vi "Bang-Bang Gain Tool.vi"() -> ()   [LabVIEW 2018]
doc: "This example demonstrates how to use Advanced PID autotuning VI where you can change the autotuning algorithm while you run the VI."
uses:
  <vilib>/DAQmx/read.llb/DAQmx Read (Analog DBL 1Chan 1Samp).vi
  <vilib>/DAQmx/write.llb/DAQmx Write (Analog DBL 1Chan 1Samp).vi
  <vilib>/DAQmx/create/channels.llb/DAQmx Create Channel (AO-Voltage-Basic).vi
  <vilib>/DAQmx/create/channels.llb/DAQmx Create Channel (AI-Temperature-Thermocouple).vi
  <vilib>/addons/control/pid/pid.llb/PID Gain Schedule (DBL).vi
  <vilib>/DAQmx/miscellaneous.llb/DAQmx Fill In Error Info.vi
  <vilib>/addons/control/pid/autopid.llb/PID Online Autotuning (Step Closed Loop).vi
  <vilib>/addons/control/pid/pid.llb/PID Advanced (DBL).vi
  <vilib>/addons/control/pid/NI_PID_autopid.lvlib
  <vilib>/addons/control/pid/NI_PID_pid.lvlib
  <vilib>/ptbypt/NI_PtbyPt.lvlib
panel:
  out "Numeric":dbl
  out "Heaters":bool
  in  "ON/OFF":bool caption="Heater Power"
  in  "Tab Control 2":enum32{"Instructions", "Plant Parameters"}(tab)
  in  "Instructions":string="Overview: This example demonstrates how to use the  PID Online Autotuning VI with the PID using the Closed-Loop Step Response Technique. This VI also shows how to handle Gain-scheduling process.\nInstructions:\n1. Run the VI and wait until the process variable (PV) reaches near setpoint (SP).\n2.  On the PID Autotuning Design section, select the type of controller and excitation amplitude for the 'closed-loop step response'. Then, click Autotune to start the process.\n3.  When the tuned PID gains do not change anymore, the identification is done and you can add a new gain by pressing Insert gains. That will also transfer the new gain to PID Gains array. Press Replace gains if you just want to substitute the previous recorded gains.\n4. Click Autotune again to go back to the automatic control. Look at the Gain Scheduling tab to see the new gain added to the list. You can change the plant to another setpoint and repeat this process to identify the gain for another operating point.\n5. Click Stop to stop the VI.\n"
  in  "Insert gains":bool
  in  "Tab Control":enum32{"PID", "Gain Scheduling"}(tab)
  out "PID Gains":T1={"proportional gain (Kc)"=6.925505792902687, "integral time (Ti, min)"=0.004930412653813362, "derivative time (Td, min)"=0.0} {"derivative time (Td, min)" format="%#.6g"; "integral time (Ti, min)" format="%#.6g"; "proportional gain (Kc)" format="%#.6g"}
  in  "SP:":dbl(slide)=10.0 min=0.0 max=0.0 scale=0.0..100.0
  in  "MV:":dbl(slide)=-7.438794336301588e-06 scale=-100.0..100.0
  out "PV:":dbl(slide)=45.098041757771064 scale=0.0..100.0
  in  "Autotune":bool
  in  "Reinitialize":bool
  in  "Automatic":bool=TRUE
  in  "alpha":dbl=nan format="%.2f"
  out "Gain Scheduling":i32
  in  "PID gain schedule":T2(array[cluster])=[{"PID gains"={"Kc"=7.0, "Ti"=0.001, "Td"=0.0}, "max value"=0.0}] {"max value" format="%.2f"; "PID gains"."Td" format="%#.3g"; "PID gains"."Ti" format="%#.3g"; "PID gains"."Kc" format="%#.3g"}
  in  "autotuning parameters":T3={"Type of Controller"=1, "relay cycles"=3, "amplitude"=1.0, "control specifications"=2, "PV noise level"=0.1} {"PV noise level" format="%.2f"; "control specifications" items=["fast", "normal", "slow"]; "amplitude" format="%.2f"; "Type of Controller" items=["P", "PI", "PID"]}
  out "MV":dbl(graph)
  in  "Replace gains":bool
  out "tuned PID gains":T1={"proportional gain (Kc)"=1.9838195929127882, "integral time (Ti, min)"=0.01995856284686879, "derivative time (Td, min)"=0.0} {"derivative time (Td, min)" format="%#.6g"; "integral time (Ti, min)" format="%#.6g"; "proportional gain (Kc)" format="%#.6g"}
  in  "Sampling Time dt (s)":dbl=0.05 min=0.001 step=0.01 format="%#.3p"
  in  "Stop":bool
  out "SP and PV":cluster{"initial PV":dbl, "SP1:":dbl}(graph)={"initial PV"=50.98160323470328, "SP1:"=50.98039215686275}
  # "PID Autotuning Design"
  # "Plant Simulated Parameters"
  # "Proportional-Integral-Derivative (PID) Controller"
  # "PID Gains"
  # "Operating Point"
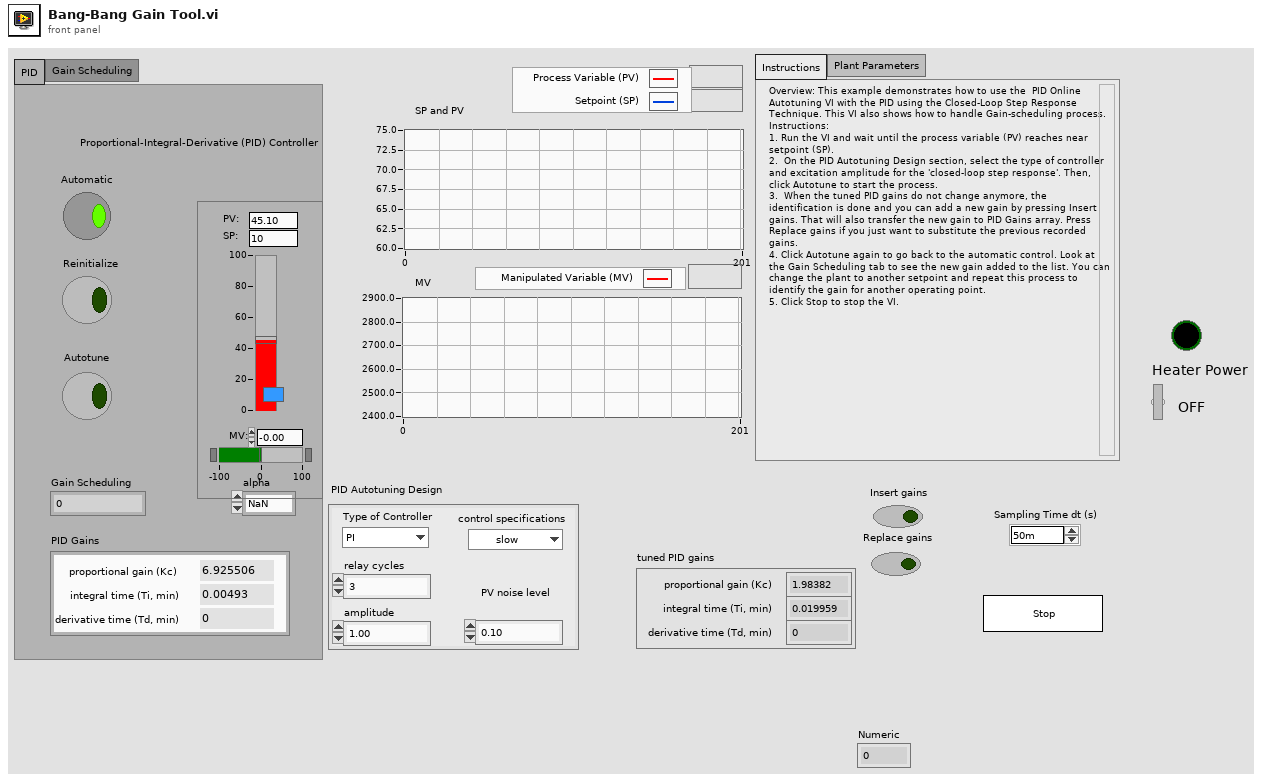
[diagram p1: front panel]
types:
  T1 = cluster{"proportional gain (Kc)":dbl, "integral time (Ti, min)":dbl, "derivative time (Td, min)":dbl}
  T2 = cluster{"PID gains":cluster{"Kc":dbl, "Ti":dbl, "Td":dbl}, "max value":dbl}[]
  T3 = cluster{"Type of Controller":u16, "relay cycles":i32, "amplitude":dbl, "control specifications":u16, "PV noise level":dbl}
  T4 = cluster{"tuned PID gains":cluster{"proportional gain (Kc)":dbl, "integral time (Ti, min)":dbl, "derivative time (Td, min)":dbl}, "SP:":dbl}
  T5 = cluster{"PID gains":cluster{"Kc":dbl, "Ti":dbl, "Td":dbl}, "max value":dbl}
  T6 = cluster{"tuned PID gains":cluster{"proportional gain (Kc)":dbl, "integral time (Ti, min)":dbl, "derivative time (Td, min)":dbl}, "max value":dbl}
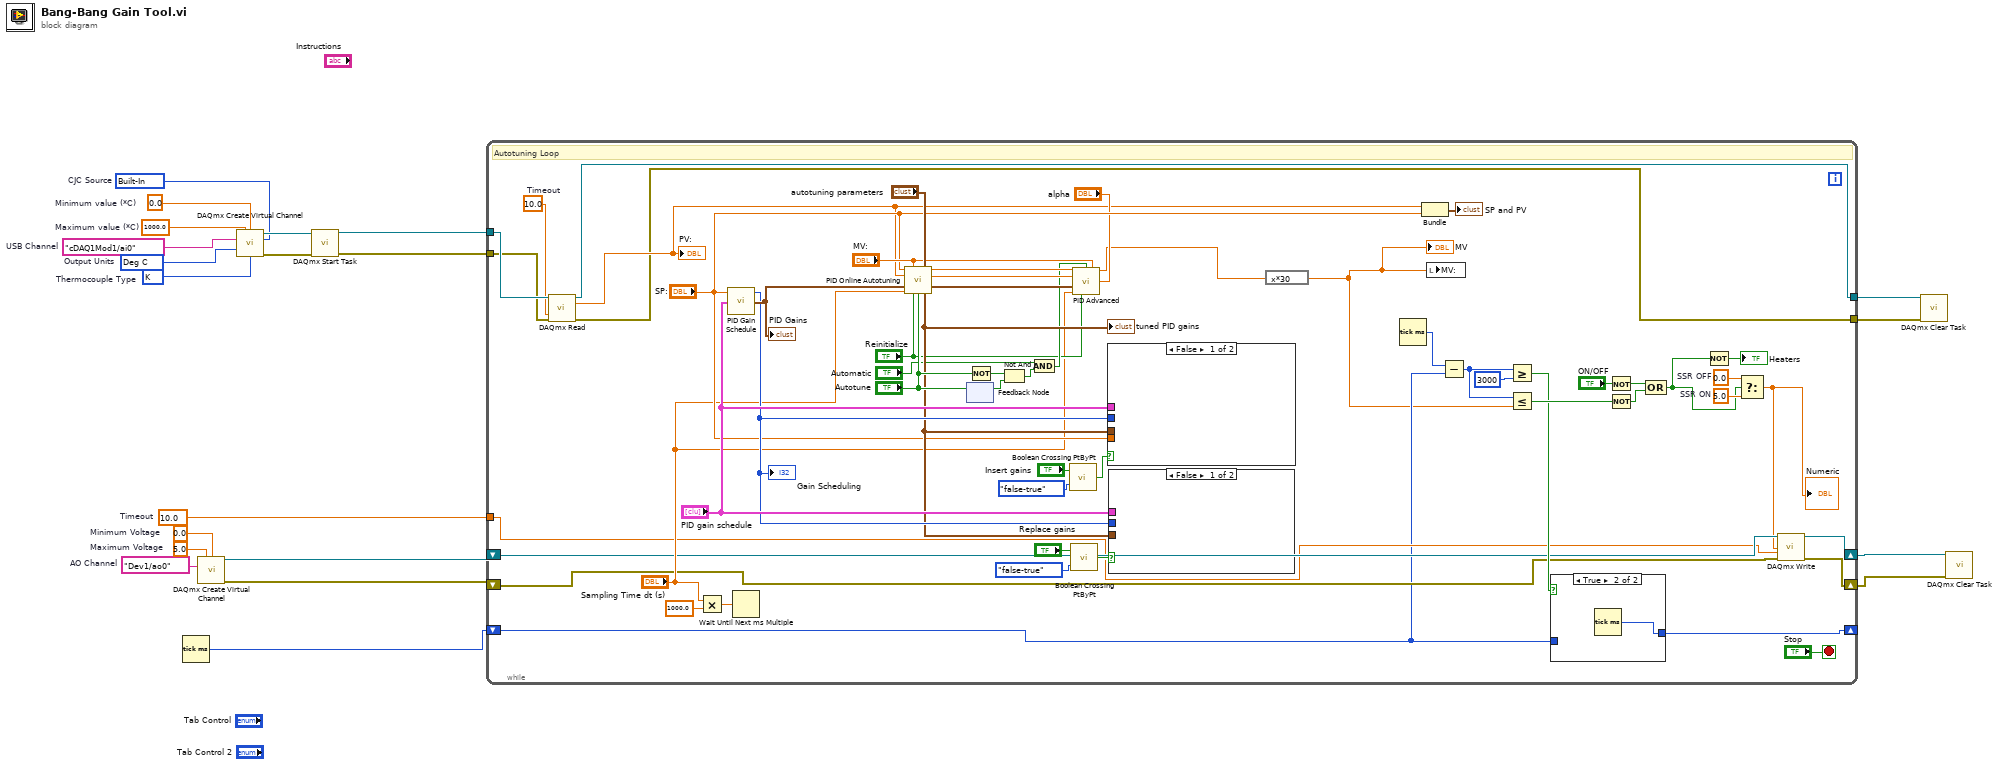
[diagram p0: block diagram]
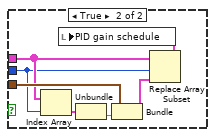
[diagram p3: hidden frame]
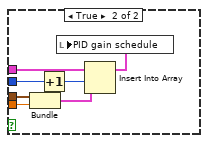
[diagram p4: hidden frame]
diagram:
  w10 = 10143 items=["Deg C"=10143, "Deg F"=10144, "Kelvins"=10325, "Deg R"=10145, "From Custom Scale"=10065]  # Output Units
  w8 = 10073 items=["J"=10072, "K"=10073, "N"=10077, "R"=10082, "S"=10085, "T"=10086, "B"=10047, "E"=10055]  # Thermocouple Type
  w9 = tag "cDAQ1Mod1/ai0"  # USB Channel
  w13 = 1000.0  # Maximum value (*C)
  w14 = 0.0  # Minimum value (*C)
  w7 = 10200 items=["Built-In"=10200, "Constant Value"=10116, "Channel"=10113]  # CJC Source
  w18 = tag "Dev1/ao0"  # AO Channel
  w19 = 5.0  # Maximum Voltage
  w20 = 0.0  # Minimum Voltage
  w15 = 10.0  # Timeout
  n1 = Tick Count (ms)() -> (millisecond timer value=w21:u32)
  n2 = call-poly <vilib>:"DAQmx Create Virtual Channel.vi"("maximum value"=w19, "minimum value"=w20, "physical channels"=w18) -> ("task out"=w17:refnum<k21>, "error out"=w16:errorcluster)  [unwired: 11 in]
  n3 = call-poly <vilib>:"DAQmx Create Virtual Channel.vi"("maximum value"=w13, "minimum value"=w14, "physical channels"=w9, "cjc source"=w7, "units"=w10, "thermocouple type"=w8) -> ("task out"=w12:refnum<k21>, "error out"=w11:errorcluster)  [unwired: 8 in]
  n4 = call <vilib>:"DAQmx Start Task.vi"("task/channels in"=w12, "error in"=w11) -> ("task out"=w6:refnum<k21>, "error out"=w5:errorcluster)  [unwired: 12 in]
  n5 = while {
    shift-right: [w38] -> _
    shift-left: w21 -> [w30]
    shift-right: [w34] -> w2
    shift-left: w17 -> [w37]
    shift-right: [w33] -> w1
    shift-left: w16 -> [w36]
    tunnel: w15 -> [w35]
    tunnel: w6 -> [w28]
    tunnel: w5 -> [w27]
    tunnel: [w25] -> w4
    tunnel: [w24] -> w3
    stop <- "Stop" stop-if-true
    w26 = 10.0  # Timeout
    w46 = 5.0  # SSR ON
    w47 = 0.0  # SSR OFF
    # "Autotuning Loop"
    n6 = call-poly <vilib>:"DAQmx Read.vi"("task/channels in"=w28, "timeout"=w26, "error in"=w27) -> ("task out"=w25:refnum<k21>, "data"=w29:dbl, "error out"=w24:errorcluster)  [unwired: 10 in]
    "PV:" <- w29
    n7 = Multiply(x="Sampling Time dt (s)", y=1000.0) -> (x*y=w55:dbl)
    n8 = call-poly <vilib>:"PID Gain Schedule.vi"("PID gain schedule"="PID gain schedule", "gain scheduling value"="SP:") -> ("PID gains out"=w65:T1, "index out"=w60:i32)  [unwired: 2 in]
    "PID Gains" <- w65
    "Gain Scheduling" <- w60
    n9 = Wait Until Next ms Multiple(millisecond multiple=w55) -> ()  [unwired: 1 out]
    n10 = call-poly <vilib>:"PID Online Autotuning.vi"("setpoint"="SP:", "manipulated variable"="MV:", "autotuning parameters"="autotuning parameters", "process variable"=w29, "PID gains in"=w65, "dt (s)"="Sampling Time dt (s)", "reinitialize? (F)"="Reinitialize", "autotune? (F)"="Autotune") -> ("setpoint out"=w76:dbl, "process variable out"=w75:dbl, "PID gains out"=w73:T1, "tuned PID gains"=w59:T1)  [unwired: 3 in, 1 out]
    "tuned PID gains" <- w59
    n11 = feedback #1() -> (w71:bool)  [unwired: 1 in]
    n12 = feedback-in #1("Autotune") -> ()
    n13 = Not(x="Autotune") -> (.not. x?=w68:bool)
    n14 = Not And(1:w71, 2:w68) -> (0:w69:bool)
    n15 = And(x="Automatic", y=w69) -> (x .and. y?=w53:bool)
    n16 = call <vilib>:"Boolean Crossing PtByPt.vi"("direction"=enum16{"either", "false-true", "true-false"}."false-true", "input"="Insert gains") -> ("crossing"=w66:bool)  [unwired: 1 in]
    n17 = call <vilib>:"Boolean Crossing PtByPt.vi"("direction"=enum16{"either", "false-true", "true-false"}."false-true", "input"="Replace gains") -> ("crossing"=w62:bool)  [unwired: 1 in]
    n18 = call-poly <vilib>:"PID Advanced.vi"("setpoint"=w76, "auto? (T)"=w53, "manual control"="MV:", "process variable"=w75, "alpha"="alpha", "PID gains"=w73, "dt (s)"="Sampling Time dt (s)", "reinitialize? (F)"="Reinitialize") -> ("output"=w23:dbl)  [unwired: 6 in, 1 out]
    n19 = case shown="False" w66 {
      tunnel: w59 -> [_ w94]
      tunnel: "SP:" -> [_ w93]
      tunnel: "PID gain schedule" -> [_ w91]
      tunnel: w60 -> [_ w89]
      frame False {
      }
      frame True {
        n20 = Bundle("tuned PID gains"=w94, "SP:"=w93) -> (w92:T4)  [unwired: 1 in]
        n21 = Increment(x=w89) -> (x+1=w88:i32)
        n22 = Insert Into Array(array=w91, index=w88, new element=w92) -> (w90:T2)
        n23 = local write "PID gain schedule"(w90) -> ()
      }
    }
    n24 = case shown="False" w62 {
      tunnel: w59 -> [_ w87]
      tunnel: "PID gain schedule" -> [_ w84]
      tunnel: w60 -> [_ w83]
      frame False {
      }
      frame True {
        n25 = Index Array(array=w84, index=w83) -> (element=w82:T5)
        n26 = Unbundle(w82) -> ("max value"=w81:dbl)  [unwired: 1 out]
        n27 = Bundle("tuned PID gains"=w87, "max value"=w81) -> (w85:T6)  [unwired: 1 in]
        n28 = Replace Array Subset(array=w84, new element=w85, index=w83) -> (w86:T2)
        n29 = local write "PID gain schedule"(w86) -> ()
      }
    }
    n30 = expression code="x*30"(w23) -> (w22:dbl)
    "MV" <- w22
    n31 = Tick Count (ms)() -> (millisecond timer value=w31:u32)
    n32 = Bundle("data"=w29, "SP:"="SP:") -> (→"SP and PV":cluster{"data":dbl, "SP:":dbl})  [unwired: 1 in]
    n33 = local write "MV:"(w22) -> ()
    n34 = Subtract(x=w31, y=w30) -> (x-y=w49:u32)
    n35 = Greater Or Equal?(x=w49, y=u32 3000) -> (x >= y?=w40:bool)
    n36 = Less Or Equal?(x=w49, y=w22) -> (x <= y?=w42:bool)
    n37 = case shown="True" w40 {
      tunnel: w30 -> [w79 _]
      tunnel: [w79 w80] -> w38
      frame False {
      }
      frame True {
        n38 = Tick Count (ms)() -> (millisecond timer value=w80:u32)
      }
    }
    n39 = Not(x="ON/OFF") -> (.not. x?=w50:bool)
    n40 = Not(x=w42) -> (.not. x?=w41:bool)
    n41 = Compound Arithmetic op=OR(w50, w41) -> (w43:bool)
    n42 = Not(x=w43) -> (.not. x?=→"Heaters":bool)
    n43 = Select(t=w47, s=w43, f=w46) -> (s? t:f=w32:dbl)
    "Numeric" <- w32
    n44 = call-poly <vilib>:"DAQmx Write.vi"("task/channels in"=w37, "data"=w32, "timeout"=w35, "error in"=w36) -> ("task out"=w34:refnum<k21>, "error out"=w33:errorcluster)  [unwired: 9 in, 1 out]
  }
  n45 = call <vilib>:"DAQmx Clear Task.vi"("task in"=w4, "error in"=w3) -> ()  [unwired: 13 in, 1 out]
  n46 = call <vilib>:"DAQmx Clear Task.vi"("task in"=w2, "error in"=w1) -> ()  [unwired: 13 in, 1 out]
